vi "niRFUtil RFHS Channelizer CreateChannelizer CSG phaseII.vi"(0 "Channelizer Spec":T3={"freq in Hz"=TRUE, "Filter Type Hint"=enum."Auto", "Hint Value"=0.0, "Channels"=[]} {"Channels"."Flags" items=["None"=0, "Force Fractional"=1, "Use Multistage"=2, "Use Pretrigger Data "=256, "Frequency Shift Only"=4]; "Channels"."fs" format="%#_8p"; "Channels"."fc" format="%#_6p"; "Channels"."stopBW" format="%#_6p"; "Channels"."passBW" format="%#_6p"; "Hint Value" format="%#_8p"}, 1 "Type":T1, 2 "Benchmark Task":T8, 3 "Replace Filter Data":bool, 5 "fs [Hz]":dbl=1000000000.0 format="%#_6p", 7 "Mode":T2, 9 "Buffer Size (s)":dbl=0.003 format="%#_6p", 11 "error in (no error)":errorcluster, 13 "User Filter Spec":T7) -> (4 "Channelizer Ref":refnum<data-value>, 15 "error out":errorcluster)   [LabVIEW 2015, in "niRFUtil.lvlib"]
uses:
  niRFUtil.lvlib
  Utilities/Benchmark/niRFUtil RFHS Benchmark Task.ctl
  Utilities/niRFUtil RFHS Util User Filter Specification.ctl
  Includes/niRFUtil RFHS Channelizer ChannelSpecification.ctl
  Includes/niRFUtil RFHS Channelizer FilterTypeHint.ctl
  Includes/niRFUtil RFHS Channelizer ChannelSpecificationBase.ctl
  Includes/niRFUtil RFHS Channelizer ChannelFlags.ctl
  Includes/niRFUtil RFHS Channelizer ChannelizerBufferingMode.ctl
  Includes/niRFUtil RFHS Channelizer ChannelizerInfo CSG.ctl
  Includes/niRFUtil RFHS Channelizer FilterRef.ctl
  Utilities/Data FIFO/niRFUtil RFHS FIFO Reference.ctl
  Utilities/Data FIFO/niRFUtil RFHS FIFO.ctl
  Includes/niRFUtil RFHS Channelizer ChannelizerType.ctl
  Includes/niRFUtil RFHS Channelizer ChannelizerFlags.ctl
  Includes/niRFUtil RFHS Channelizer FilterSpecification.ctl
panel:
  in  "Inital Phase":dbl
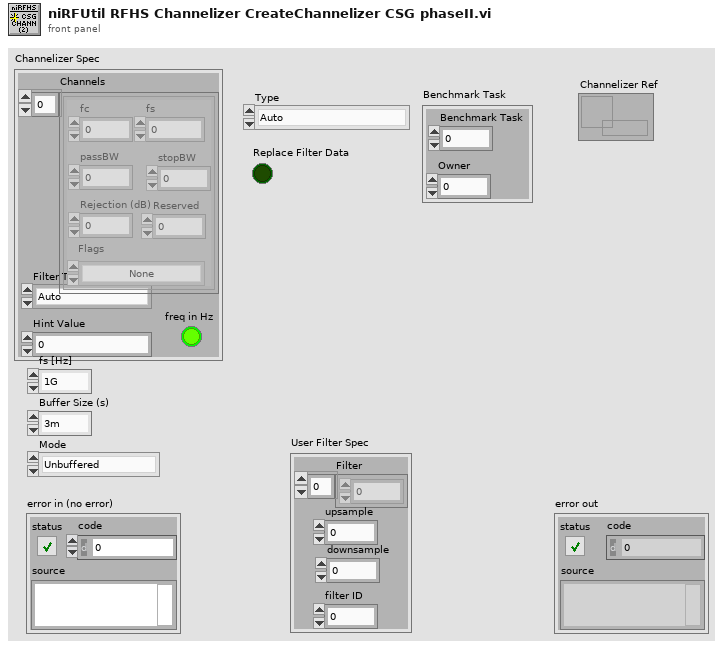
[diagram p1: front panel]
types:
  T1 = typedef "niRFUtil.lvlib/niRFUtil RFHS Channelizer ChannelizerType.ctl" = enum32{"Auto", "Frequency Shift Only", "Resampler Only"}
  T2 = typedef "niRFUtil.lvlib/niRFUtil RFHS Channelizer ChannelizerBufferingMode.ctl" = enum32{"Unbuffered", "Finite", "Continuous"}
  T3 = typedef "niRFUtil.lvlib/niRFUtil RFHS Channelizer ChannelSpecification.ctl" = cluster{"freq in Hz":bool, "Filter Type Hint":T4, "Hint Value":dbl, "Channels":T5[]}
  T4 = typedef "niRFUtil.lvlib/niRFUtil RFHS Channelizer FilterTypeHint.ctl" = enum16{"Auto", "FFT (LTE)", "FFT (WiFi)", "FFT (custom)"}
  T5 = typedef "niRFUtil.lvlib/niRFUtil RFHS Channelizer ChannelSpecificationBase.ctl" = cluster{"fc":dbl, "fs":dbl, "passBW":dbl, "stopBW":dbl, "Rejection (dB)":dbl, "Flags":T6, "Reserved":i32}
  T6 = typedef "niRFUtil.lvlib/niRFUtil RFHS Channelizer ChannelFlags.ctl" = u32
  T7 = typedef "niRFUtil.lvlib/niRFUtil RFHS Util User Filter Specification.ctl" = cluster{"Filter":dbl[], "upsample":i32, "downsample":i32, "filter ID":i32}
  T8 = typedef "niRFUtil.lvlib/niRFUtil RFHS Benchmark Task.ctl" = cluster{"Benchmark Task":u64, "Owner":u32}
  T9 = typedef "niRFUtil.lvlib/niRFUtil RFHS Channelizer ChannelizerInfo CSG.ctl" = cluster{"Filter LVRef":T10, "Mode":T2, "History":csg[], "Buffer":csg[], "FIFO":T11, "History Len":u32, "Float Cache":csg[], "Double Cache":cdb[], "Type":T1, "Resample Phase":dbl, "fft1Descriptors":u64[], "fft2Descriptors":u64[], "FFT tBuf":csg[], "guardBandLen":i32, "FFT History":csg[], "FFT History Len":u32, "FFTInitDone":u32, "FFT Filter LVRefs":T10[], "FFT fc Offs":u32[], "fft2Sizes":u32[], "BufferW":u32[], "BufferR":u32[], "Buff Off":u32[], "Phase0 (fshift)":dbl[], "Phase (fshift)":dbl[], "fs phase step":dbl[], "Resample Step":dbl, "Flags":T13, "Reset Cnt":i64, "Filter Pass":u32, "Stages":variant[]}
  T10 = typedef "niRFUtil.lvlib/niRFUtil RFHS Channelizer FilterRef.ctl" = cluster{"Ref":u64, "GUID":u64, "Upsample":i32, "Downsample":i32, "Size":i32, "Num Taps":i32}
  T11 = typedef "niRFUtil.lvlib/niRFUtil RFHS FIFO Reference.ctl" = cluster{"Read Lock":refnum<data-value>, "Info":T12, "Write Lock":refnum<data-value>}
  T12 = typedef "niRFUtil.lvlib/niRFUtil RFHS FIFO.ctl" = cluster{"ID":u64, "Length":u32}
  T13 = typedef "niRFUtil.lvlib/niRFUtil RFHS Channelizer ChannelizerFlags.ctl" = u32
  T14 = enum32{"Reserved", "Rational", "Fine Tune", "Fractional", "Rational (user)", "Reserved 2", "Fractional (user)", "FFT Resampler"}
  T15 = typedef "niRFUtil.lvlib/niRFUtil RFHS Channelizer FilterSpecification.ctl" = cluster{"Type":enum32{"Reserved", "Rational", "Fine Tune", "Fractional", "Rational (user)", "Reserved 2", "Fractional (user)", "FFT Resampler"}, "Reserved":i32, "Spec":T5}
  T16 = enum32{"Reserved", "Rational", "Fine Tune", "Fractional", "Rational (user)", "Reserved 2", "Fractional (user)"}
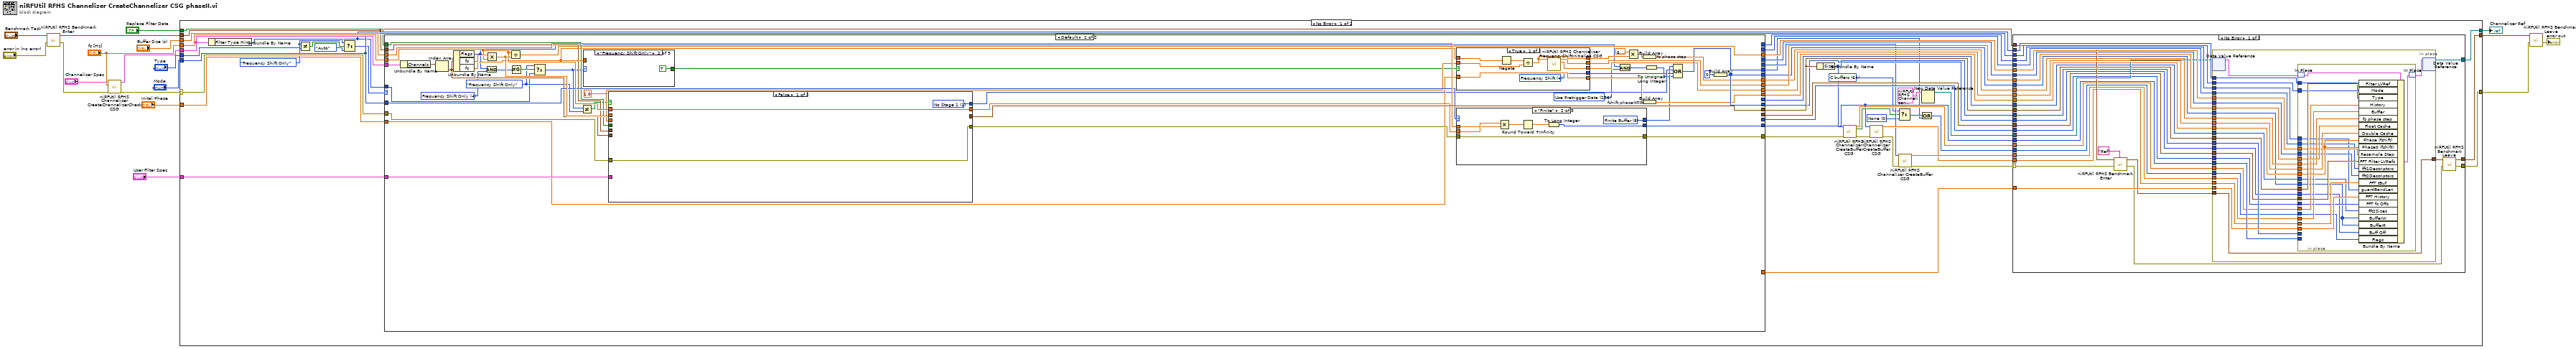
[diagram p0: block diagram]
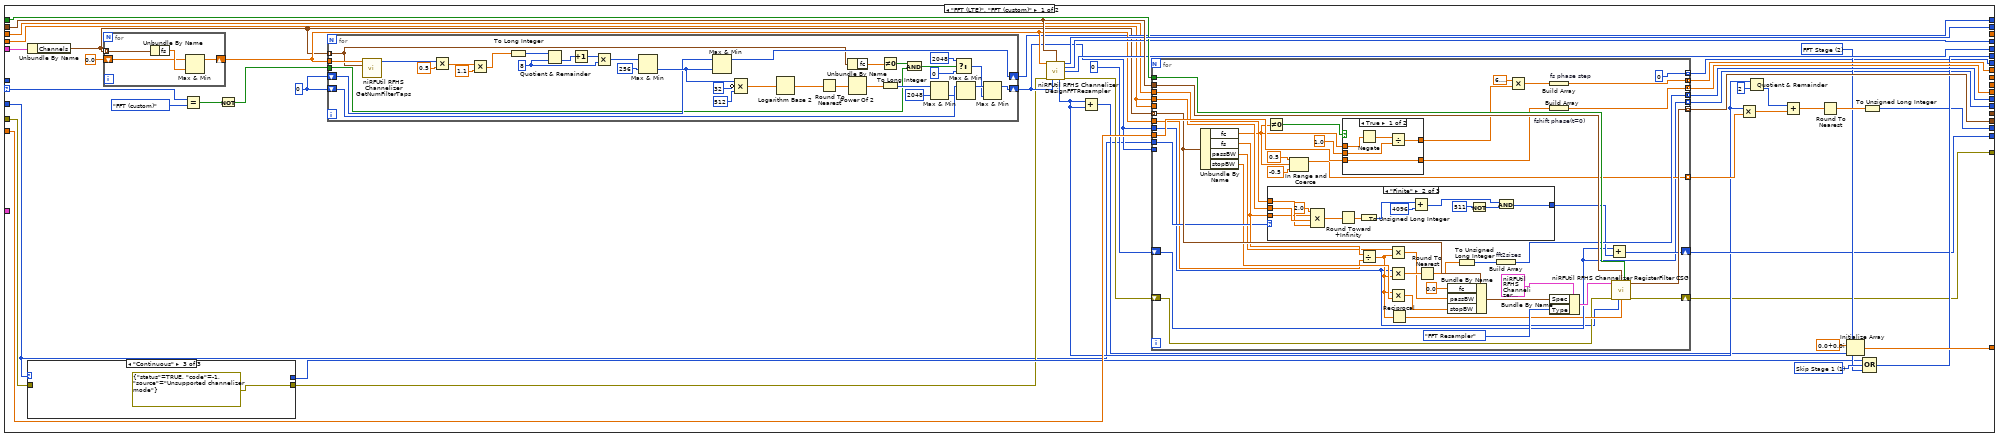
[diagram p3: hidden frame]
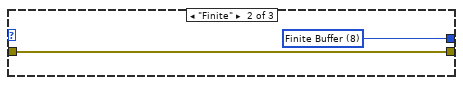
[diagram p8: hidden frame]
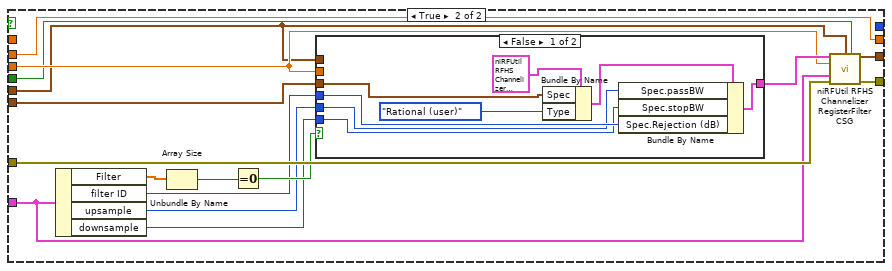
[diagram p10: hidden frame]
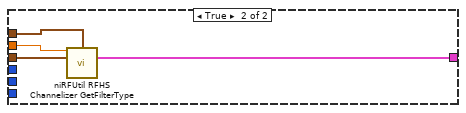
[diagram p11: hidden frame]
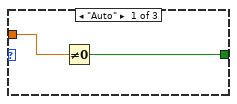
[diagram p12: hidden frame]
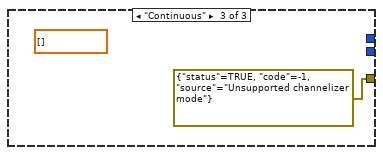
[diagram p15: hidden frame]
diagram:
  n1 = call "niRFUtil RFHS Benchmark Enter.vi"("error in (no error)"="error in (no error)", "Benchmark Task (Parent)"="Benchmark Task") -> ("error out"=w5:errorcluster, "Benchmark Task (Self)"=w7:T8)  [unwired: 8 in]
  n2 = call "niRFUtil RFHS Channelizer CreateChannelizerCheck CSG.vi"("Channel Spec"="Channelizer Spec", "fs [Hz]"="fs [Hz]", "error in (no error)"=w5) -> ("Channel Spec (out)"=w1:T3, "error out"=w4:errorcluster)  [unwired: 11 in]
  n3 = case shown="No Error" w4 {
    selector: w4 -> [w69 w404]
    tunnel: [w37 w404] -> w17
    tunnel: w1 -> [w19 _]
    tunnel: "fs [Hz]" -> [w62 _]
    tunnel: "User Filter Spec" -> [w68 _]
    tunnel: "Mode" -> [w61 _]
    tunnel: "Type" -> [w55 _]
    tunnel: w7 -> [w20 w403]
    tunnel: [w48 _] -> w11
    tunnel: "Buffer Size (s)" -> [w66 _]
    tunnel: "Inital Phase" -> [w43 _]
    tunnel: "Replace Filter Data" -> [w53 _]
    tunnel: [w47 w403] -> w6
    frame No Error {
      w22 = T13 64 items=["None"=0, "Skip Stage 1"=1, "FFT Stage"=2, "Frequency Shift"=4, "Finite Buffer"=8, "Reset"=16, "Input Len Estimate"=32, "C buffers"=64] ("t")
      w23 = T13 0 items=["None"=0, "Skip Stage 1"=1, "FFT Stage"=2, "Frequency Shift"=4, "Finite Buffer"=8, "Reset"=16, "Input Len Estimate"=32] ("Flags")
      n4 = Unbundle By Name(w19) -> ("Filter Type Hint"=w59:T4)
      n5 = Not Equal?(x=w55, y=niRFUtil_RFHS_Channelizer_ChannelizerType."Frequency Shift Only") -> (x != y?=w54:bool)
      n6 = Select(t=w59, s=w54, f=niRFUtil_RFHS_Channelizer_FilterTypeHint."Auto") -> (s? t:f=w40:T4)
      n7 = case shown="Default" w40 {
        selector: w40 -> [w159 _]
        tunnel: w69 -> [w154 w351]
        tunnel: w68 -> [_ w350]
        tunnel: [_ w349] -> w67
        tunnel: [w162 w347] -> w36
        tunnel: w66 -> [w173 w346]
        tunnel: [_ w318] -> w65
        tunnel: [_ w317] -> w64
        tunnel: [_ w325] -> w63
        tunnel: w62 -> [w172 w342]
        tunnel: w19 -> [w182 w326]
        tunnel: w61 -> [w161 w341]
        tunnel: w20 -> [w200 w340]
        tunnel: [w199 _] -> w58
        tunnel: [w198 _] -> w57
        tunnel: [w176 _] -> w56
        tunnel: w55 -> [_ w307]
        tunnel: w53 -> [w197 w339]
        tunnel: [w196 _] -> w52
        tunnel: [w169 w338] -> w32
        tunnel: [w195 _] -> w27
        tunnel: [w174 _] -> w46
        tunnel: [w194 _] -> w38
        tunnel: [w168 w332] -> w45
        tunnel: [w193 _] -> w39
        tunnel: [w170 w332] -> w44
        tunnel: w43 -> [w192 w335]
        tunnel: [w184 w330] -> w42
        tunnel: [w183 w328] -> w41
        tunnel: [w179 w319] -> w24
        frame "FFT (LTE)", "FFT (custom)" {
          w156 = 0
          w180 = T13 2 items=["None"=0, "Skip Stage 1"=1, "FFT Stage"=2, "Frequency Shift"=4] ("Flags")
          w181 = T13 1 items=["None"=0, "Skip Stage 1"=1, "FFT Stage"=2, "Frequency Shift"=4] ("Flags")
          n8 = Unbundle By Name(w182) -> ("Channels"=w155:T5[])
          n9 = case shown="\"Continuous\"" w161 {
            tunnel: w154 -> [w301 w303 _]
            tunnel: [w301 w303 errorcluster {"status"=TRUE, "code"=-1, "source"="Unsupported channelizer mode"} ("error out")] -> w164
            tunnel: [_ w302 _] -> w167
            frame "Unbuffered" {
            }
            frame "Finite" {
              w302 = T13 8 items=["None"=0, "Skip Stage 1"=1, "FFT Stage"=2, "Frequency Shift"=4, "Finite Buffer"=8] ("Flags")
            }
            frame "Continuous" {
            }
          }
          n10 = for {
            tunnel: w155 -> [w265] mode=indexing
            shift-right: [w263] -> w177
            shift-left: 0.0 -> [w262]
            n11 = Unbundle By Name(w265) -> ("fs"=w264:dbl)
            n12 = Max & Min(x=w262, y=w264) -> (max(x,y)=w263:dbl)  [unwired: 1 out]
          }
          n13 = Equal?(x=w159, y=niRFUtil_RFHS_Channelizer_FilterTypeHint."FFT (custom)") -> (x = y?=w158:bool)
          n14 = Not(x=w158) -> (.not. x?=w157:bool)
          n15 = for {
            tunnel: w155 -> [w275] mode=indexing
            shift-right: [w266] -> w175
            shift-left: w156 -> [w282]
            tunnel: w177 -> [w281]
            shift-right: [w277] -> w176
            shift-left: w156 -> [w278]
            tunnel: w157 -> [w272]
            w291 = 8 ("y")
            n16 = call "niRFUtil RFHS Channelizer GetNumFilterTaps.vi"("fs"=w281, "Channel Specification"=w275) -> ("#Filter Taps"=w280:i32)  [unwired: 13 in]
            n17 = Multiply(x=w280, y=0.5) -> (x*y=w284:dbl)
            n18 = Multiply(x=w284, y=1.1) -> (x*y=w286:dbl)
            n19 = To Long Integer(number=w286) -> (32bit integer=w288:i32)
            n20 = Quotient & Remainder(x=w288, y=w291) -> (floor(x/y)=w289:i32)  [unwired: 1 out]
            n21 = Increment(x=w289) -> (x+1=w290:i32)
            n22 = Multiply(x=w290, y=w291) -> (x*y=w292:i32)
            n23 = Max & Min(x=w292, y=256) -> (min(x,y)=w279:i32)  [unwired: 1 out]
            n24 = Max & Min(x=w278, y=w279) -> (max(x,y)=w277:i32)  [unwired: 1 out]
            n25 = Compound Arithmetic op=MULTIPLY(w279, invert 32 ("value"), 512 ("value")) -> (w295:dbl)
            n26 = Logarithm Base 2(1:w295) -> (0:w296:dbl)
            n27 = Round To Nearest(number=w296) -> (nearest integer value=w297:dbl)
            n28 = Unbundle By Name(w275) -> ("fc"=w274:dbl)
            n29 = Power Of 2(x=w297) -> (2^x=w298:dbl)
            n30 = Not Equal To 0?(x=w274) -> (x != 0?=w273:bool)
            n31 = To Long Integer(number=w298) -> (32bit integer=w299:i32)
            n32 = And(x=w273, y=w272) -> (x .and. y?=w270:bool)
            n33 = Max & Min(x=w299, y=2048) -> (min(x,y)=w276:i32)  [unwired: 1 out]
            n34 = Select(t=2048 ("Len Hint"), s=w270, f=0 ("Len Hint")) -> (s? t:f=w267:i32)
            n35 = Max & Min(x=w282, y=w276) -> (max(x,y)=w268:i32)  [unwired: 1 out]
            n36 = Max & Min(x=w268, y=w267) -> (max(x,y)=w266:i32)  [unwired: 1 out]
          }
          n37 = call "niRFUtil RFHS Channelizer DesignFFTResampler.vi"("Channel fs"=w177, "Benchmark Task"=w200, "error in (no error)"=w164, "fft2Size"=w175) -> ("fft1Descriptors"=w198:u64[], "fft2Descriptors"=w193:u64[], "Buffer Size"=w195:i32, "fft1Size"=w166:i32, "error out"=w163:errorcluster)  [unwired: 7 in]
          n38 = Add(x=w166, y=w166) -> (x+y=w165:i32)
          n39 = for {
            tunnel: w200 -> [w243]
            tunnel: [w224] -> w199 mode=indexing
            tunnel: w197 -> [w242]
            tunnel: [w241] -> w194 mode=concatenating
            tunnel: w192 -> [w239]
            tunnel: [w223] -> w185 mode=indexing
            tunnel: [w230] -> w184 mode=concatenating
            tunnel: [w229] -> w183 mode=concatenating
            tunnel: w155 -> [w228] mode=indexing
            tunnel: w172 -> [_]
            tunnel: w175 -> [w202]
            tunnel: w177 -> [w208]
            tunnel: w175 -> [_]
            tunnel: w173 -> [w220]
            tunnel: w172 -> [w219]
            tunnel: w161 -> [w217]
            tunnel: [w214] -> w170 mode=indexing
            shift-right: [w216] -> w169
            shift-left: u32 0 -> [w214]
            tunnel: [u32 0] -> w168 mode=indexing
            shift-right: [w204] -> w162
            shift-left: w163 -> [w205]
            n40 = Unbundle By Name(w228) -> ("fc"=w201:dbl, "fs"=w218:dbl, "passBW"=w212:dbl, "stopBW"=w210:dbl)
            n41 = Not Equal To 0?(x=w201) -> (x != 0?=w203:bool)
            n42 = case shown="\"Finite\"" w217 {
              tunnel: w220 -> [_ w255 _]
              tunnel: w219 -> [_ w256 _]
              tunnel: [_ w247 _] -> w215
              tunnel: w218 -> [_ w252 _]
              frame "Unbuffered" {
              }
              frame "Finite" {
                n43 = Compound Arithmetic op=MULTIPLY(2.0 ("value"), w252, w256, w255) -> (w254:dbl)
                n44 = Round Toward +Infinity(x=w254) -> (ceil(x): smallest int >= x=w253:dbl)
                n45 = To Unsigned Long Integer(number=w253) -> (unsigned 32bit integer=w251:u32)
                n46 = Add(x=w251, y=u32 4096) -> (x+y=w249:u32)
                n47 = Not(x=u32 511 ("y")) -> (.not. x?=w246:u32)
                n48 = And(x=w249, y=w246) -> (x .and. y?=w247:u32)
              }
              frame "Continuous" {
              }
            }
            n49 = In Range and Coerce(upper limit=0.5, x=w201, lower limit=-0.5) -> (coerced(x)=w223:dbl)  [unwired: 1 out]
            n50 = case shown="True" w203 {
              tunnel: [w260 _] -> w227
              tunnel: 1.0 ("t") -> [w261 _]
              tunnel: w239 -> [w259 _]
              tunnel: [w259 _] -> w231
              tunnel: w201 -> [w258 _]
              frame True {
                n51 = Negate(x=w258) -> (-x=w257:dbl)
                n52 = Divide(x=w257, y=w261) -> (x/y=w260:dbl)
              }
              frame False {
              }
            }
            n53 = Divide(x=w218, y=w208) -> (x/y=w207:dbl)
            n54 = Multiply(x=w212, y=w207) -> (x*y=w211:dbl)
            n55 = Multiply(x=w202, y=w207) -> (x*y=w222:dbl)
            n56 = Multiply(x=w207, y=w210) -> (x*y=w209:dbl)
            n57 = Reciprocal(x=w207) -> (1/x=w206:dbl)
            n58 = Round To Nearest(number=w222) -> (nearest integer value=w221:dbl)
            n59 = Bundle By Name(cluster=w228, "fc"=0.0, "passBW"=w211, "stopBW"=w209) -> (w244:T5)
            n60 = To Unsigned Long Integer(number=w221) -> (unsigned 32bit integer=w235:u32)
            n61 = Build Array "fft2sizes"(w235) -> (w241:u32[])
            n62 = Multiply(x=6.283185307179586, y=w227) -> (x*y=w225:dbl)
            n63 = Build Array "fs phase step"(w225) -> (w229:dbl[])
            n64 = Build Array "fshift phase(t=0)"(w231) -> (w230:dbl[])
            n65 = Bundle By Name(cluster=T15 {"Type"=enum."Rational", "Reserved"=0, "Spec"={"fc"=0.0, "fs"=0.0, "passBW"=0.0, "stopBW"=0.0, "Rejection (dB)"=0.0, "Flags"=0, "Reserved"=0}} ("Filter Spec"), "Spec"=w244, "Type"=T14."FFT Resampler") -> (w236:T15)
            n66 = Add(x=w214, y=w215) -> (x+y=w216:u32)
            n67 = call "niRFUtil RFHS Channelizer RegisterFilter CSG.vi"("Filter Spec"=w236, "Benchmark Task"=w243, "Replace Filter Data"=w242, "error in (no error)"=w205, "Len Hint"=w202, "Filter Scaling"=w206) -> ("Filter LVRef"=w224:T10, "error out"=w204:errorcluster)  [unwired: 8 in]
          }
          n68 = Multiply(x=w166, y=w185) -> (x*y=w188:dbl[])
          n69 = Quotient & Remainder(x=w166, y=2) -> (floor(x/y)=w189:i32)  [unwired: 1 out]
          n70 = Add(x=w189, y=w188) -> (x+y=w187:dbl[])
          n71 = Round To Nearest(number=w187) -> (nearest integer value=w186:dbl[])
          n72 = Initialize Array(csg 0.0+0.0i ("element"), w165) -> (w196:csg[])
          n73 = Compound Arithmetic op=OR(w167, w181, w180) -> (w179:T13)
          n74 = To Unsigned Long Integer(number=w186) -> (unsigned 32bit integer=w174:u32[])
        }
        frame Default {
          w311 = T6 4 items=["None"=0, "Force Fractional"=1, "Use Multistage"=2, "Use Pretrigger Data "=256, "Frequency Shift Only"=4] ("y")
          w315 = T6 256 items=["None"=0, "Force Fractional"=1, "Use Multistage"=2, "Use Pretrigger Data "=256] ("y")
          w308 = niRFUtil_RFHS_Channelizer_ChannelizerType."Frequency Shift Only" ("y")
          w337 = 1.0 ("t")
          n75 = Unbundle By Name(w326) -> ("Channels"=w327:T5[])
          n76 = Index Array(array=w327) -> (element=w312:T5)  [unwired: 1 in]
          n77 = Unbundle By Name(w312) -> ("Flags"=w305:T6, "fs"=w345:dbl, "fc"=w336:dbl)
          n78 = And(x=w305, y=w311) -> (x .and. y?=w310:T6)
          n79 = Multiply(x=w345, y=w342) -> (x*y=w343:dbl)
          n80 = Divide(x=w342, y=w343) -> (x/y=w325:dbl)
          n81 = Not Equal To 0?(x=w310) -> (x != 0?=w309:bool)
          n82 = Select(t=w308, s=w309, f=w307) -> (s? t:f=w306:T1)
          n83 = Not Equal?(x=w306, y=w308) -> (x != y?=w331:bool)
          n84 = case shown="\"Frequency Shift Only\"" w306 {
            tunnel: [w392 TRUE _] -> w329
            tunnel: w336 -> [w391 _ _]
            frame "Auto" {
              n85 = Not Equal To 0?(x=w391) -> (x != 0?=w392:bool)
            }
            frame "Frequency Shift Only" {
            }
            frame "Resampler Only" {
            }
          }
          n86 = case shown="False" w331 {
            tunnel: w351 -> [w362 w378]
            tunnel: w350 -> [_ w372]
            tunnel: [_ w377] -> w349
            tunnel: [w362 w376] -> w348
            tunnel: w340 -> [_ w363]
            tunnel: w312 -> [_ w374]
            tunnel: w337 -> [_ w367]
            tunnel: w343 -> [_ w375]
            tunnel: [w361 w375] -> w344
            tunnel: w342 -> [w361 _]
            tunnel: w339 -> [_ w364]
            tunnel: [w360 _] -> w321
            frame False {
              w360 = T13 1 items=["None"=0, "No Stage 1"=1, "FFT Stage"=2, "Frequency Shift"=4] ("Flags")
            }
            frame True {
              n87 = Unbundle By Name(w372) -> ("Filter"=w371:dbl[], "filter ID"=w368:i32, "upsample"=w366:i32, "downsample"=w365:i32)
              n88 = Array Size(array=w371) -> (size(s)=w370:i32)
              n89 = Equal To 0?(x=w370) -> (x = 0?=w369:bool)
              n90 = case shown="False" w369 {
                tunnel: w374 -> [w385 w390]
                tunnel: [w382 w389] -> w373
                tunnel: w367 -> [_ w388]
                tunnel: w368 -> [w381 _]
                tunnel: w366 -> [w380 _]
                tunnel: w365 -> [w379 _]
                tunnel: w363 -> [_ w387]
                frame False {
                  n91 = Bundle By Name(cluster=T15 {"Type"=enum."Reserved", "Reserved"=0, "Spec"={"fc"=0.0, "fs"=0.0, "passBW"=0.0, "stopBW"=0.0, "Rejection (dB)"=0.0, "Flags"=0, "Reserved"=0}} ("Filter Spec"), "Spec"=w385, "Type"=T16."Rational (user)") -> (w383:T15)
                  n92 = Bundle By Name(cluster=w383, "Spec.passBW"=w380, "Spec.stopBW"=w379, "Spec.Rejection (dB)"=w381) -> (w382:T15)
                }
                frame True {
                  n93 = call "niRFUtil RFHS Channelizer GetFilterType.vi"("fs"=w388, "Benchmark Task"=w387, "Channel Specification"=w390) -> ("Filter Spec"=w389:T15)  [unwired: 9 in, 3 out]
                }
              }
              n94 = call "niRFUtil RFHS Channelizer RegisterFilter CSG.vi"("Filter Spec"=w373, "Benchmark Task"=w363, "Replace Filter Data"=w364, "fs"=w367, "User Filter Spec"=w372, "error in (no error)"=w378) -> ("Filter LVRef"=w377:T10, "error out"=w376:errorcluster)  [unwired: 8 in]
            }
          }
          n95 = case shown="True" w329 {
            tunnel: [w354 _] -> w323
            tunnel: w337 -> [w359 _]
            tunnel: w335 -> [w358 _]
            tunnel: [w358 _] -> w334
            tunnel: w336 -> [w357 _]
            tunnel: [w355 _] -> w320
            tunnel: [w353 _] -> w318
            tunnel: [w352 _] -> w317
            frame True {
              w355 = T13 4 items=["None"=0, "No Stage 1"=1, "FFT Stage"=2, "Frequency Shift"=4] ("Flags")
              n96 = Negate(x=w357) -> (-x=w356:dbl)
              n97 = Divide(x=w356, y=w359) -> (x/y=w354:dbl)
              n98 = call "niRFUtil RFHS Channelizer FrequencyShiftInitialize CSG.vi"("fc"=w354) -> ("Float Cache"=w353:csg[], "Double Cache"=w352:cdb[])  [unwired: 13 in]
            }
            frame False {
            }
          }
          n99 = case shown="\"Finite\"" w341 {
            tunnel: w348 -> [w394 w401 _]
            tunnel: [w394 w401 errorcluster {"status"=TRUE, "code"=-1, "source"="Unsupported channelizer mode"} ("error out")] -> w347
            tunnel: w346 -> [_ w399 _]
            tunnel: w344 -> [_ w400 _]
            tunnel: [_ w396 _] -> w338
            tunnel: [_ w395 _] -> w316
            frame "Unbuffered" {
            }
            frame "Finite" {
              w395 = T13 8 items=["None"=0, "Skip Stage 1"=1, "FFT Stage"=2, "Frequency Shift"=4, "Finite Buffer"=8] ("Flags")
              n100 = Multiply(x=w400, y=w399) -> (x*y=w398:dbl)
              n101 = Round Toward +Infinity(x=w398) -> (ceil(x): smallest int >= x=w397:dbl)
              n102 = To Long Integer(number=w397) -> (32bit integer=w396:i32)
            }
            frame "Continuous" {
              (unwired) csg[] []
            }
          }
          n103 = And(x=w305, y=w315) -> (x .and. y?=w314:T6)
          n104 = Multiply(x=6.283185307179586, y=w323) -> (x*y=w322:dbl)
          n105 = Build Array "fs phase step"(w322) -> (w328:dbl[])
          n106 = Build Array "fshift phase(t=0)"(w334) -> (w330:dbl[])
          n107 = To Unsigned Long Integer(number=w314) -> (unsigned 32bit integer=w313:T6)
          n108 = Compound Arithmetic op=OR(w316, w321, w320, w313) -> (w319:T13)
          n109 = Build Array(u32 0) -> (w332:u32[])
        }
      }
      n110 = Unbundle By Name(w67) -> ("Size"=w35:i32)
      n111 = call "niRFUtil RFHS Channelizer CreateBuffer CSG.vi"("Size"=w35, "error in (no error)"=w36) -> ("Buffer"=w34:csg[], "Embedded?"=w26:bool, "error out"=w33:errorcluster)  [unwired: 11 in]
      n112 = call "niRFUtil RFHS Channelizer CreateBuffer CSG.vi"("Size"=w32, "error in (no error)"=w33) -> ("Buffer"=w31:csg[], "error out"=w30:errorcluster)  [unwired: 11 in, 1 out]
      n113 = Select(t=w22, s=w26, f=w23) -> (s? t:f=w25:T13)
      n114 = call "niRFUtil RFHS Channelizer CreateBuffer CSG.vi"("Size"=w27, "error in (no error)"=w30) -> ("Buffer"=w28:csg[], "error out"=w29:errorcluster)  [unwired: 11 in, 1 out]
      n115 = Or(x=w25, y=w24) -> (x .or. y?=w21:T13)
      n116 = New Data Value Reference(data value=T9 {"Filter LVRef"={"Ref"=0, "GUID"=0, "Upsample"=0, "Downsample"=0, "Size"=0, "Num Taps"=0}, "Mode"=enum."Unbuffered", "History"=[], "Buffer"=[], "FIFO"={"Read Lock"=refnum, "Info"={"ID"=0, "Length"=0}, "Write Lock"=refnum}, "History Len"=0, "Float Cache"=[], "Double Cache"=[], "Type"=enum."Auto", "Resample Phase"=0.0, "fft1Descriptors"=[], "fft2Descriptors"=[], "FFT tBuf"=[], "guardBandLen"=0, "FFT History"=[], "FFT History Len"=0, "FFTInitDone"=0, "FFT Filter LVRefs"=[], "FFT fc Offs"=[], "fft2Sizes"=[], "BufferW"=[], "BufferR"=[], "Buff Off"=[], "Phase0 (fshift)"=[], "Phase (fshift)"=[], "fs phase step"=[], "Resample Step"=0.0, "Flags"=0, "Reset Cnt"=0, "Filter Pass"=0, "Stages"=[]} ("Info")) -> (data value reference=w49:refnum<data-value>)  [unwired: 1 in, 1 out]
      n117 = case shown="No Error" w29 {
        selector: w29 -> [w72 w152]
        tunnel: w67 -> [w102 _]
        tunnel: w65 -> [w101 _]
        tunnel: w64 -> [w100 _]
        tunnel: w63 -> [w99 _]
        tunnel: w61 -> [w98 _]
        tunnel: w58 -> [w97 _]
        tunnel: w57 -> [w96 _]
        tunnel: w56 -> [w95 _]
        tunnel: w55 -> [w94 _]
        tunnel: w52 -> [w93 _]
        tunnel: w49 -> [w92 _]
        tunnel: [w91 _] -> w48
        tunnel: w20 -> [w90 w153]
        tunnel: [w89 w153] -> w47
        tunnel: w35 -> [w88 _]
        tunnel: w34 -> [w87 _]
        tunnel: w32 -> [w86 _]
        tunnel: w31 -> [w85 _]
        tunnel: w28 -> [w84 _]
        tunnel: w46 -> [w83 _]
        tunnel: w45 -> [w82 _]
        tunnel: w44 -> [w81 _]
        tunnel: w42 -> [w80 _]
        tunnel: w41 -> [w79 _]
        tunnel: w39 -> [w78 _]
        tunnel: w38 -> [w77 _]
        tunnel: w21 -> [w76 _]
        tunnel: [w70 w152] -> w37
        frame No Error {
          n118 = call "niRFUtil RFHS Benchmark Enter.vi"("ID"="Ref", "error in (no error)"=w72, "Benchmark Task (Parent)"=w90) -> ("error out"=w71:errorcluster, "Benchmark Task (Self)"=w74:T8)  [unwired: 7 in]
          n119 = in-place {
            in-place-border: w102 -> [w128]
            in-place-border: w101 -> [w127]
            in-place-border: w100 -> [w126]
            in-place-border: w79 -> [w125]
            in-place-border: w80 -> [w124]
            in-place-border: w99 -> [w123]
            in-place-border: w98 -> [w122]
            in-place-border: w97 -> [w121]
            in-place-border: w96 -> [w120]
            in-place-border: w78 -> [w119]
            in-place-border: w95 -> [w118]
            in-place-border: w94 -> [w117]
            in-place-border: w93 -> [w116]
            in-place-border: [w115] -> w73
            in-place-border: w74 -> [w115]
            in-place-border: w88 -> [w112]
            in-place-border: w86 -> [w111]
            in-place-border: w85 -> [w110]
            in-place-border: w87 -> [w109]
            in-place-border: w84 -> [w108]
            in-place-border: w83 -> [w107]
            in-place-border: w77 -> [w106]
            in-place-border: w82 -> [w105]
            in-place-border: w81 -> [w104]
            in-place-border: w76 -> [w103]
            n120 = in-place-dvr #1(w92) -> (w114:T9)  [unwired: 1 out]
            n121 = in-place {
              in-place-border: w128 -> [w151]
              in-place-border: w127 -> [w150]
              in-place-border: w126 -> [w149]
              in-place-border: w125 -> [w148]
              in-place-border: w124 -> [w147]
              in-place-border: w123 -> [w146]
              in-place-border: w122 -> [w145]
              in-place-border: w121 -> [w144]
              in-place-border: w120 -> [w143]
              in-place-border: w119 -> [w142]
              in-place-border: w118 -> [w141]
              in-place-border: w117 -> [w140]
              in-place-border: w116 -> [w139]
              in-place-border: w112 -> [_]
              in-place-border: w111 -> [_]
              in-place-border: w110 -> [w136]
              in-place-border: w109 -> [w135]
              in-place-border: w108 -> [w134]
              in-place-border: w107 -> [w133]
              in-place-border: w106 -> [w132]
              in-place-border: w105 -> [w131]
              in-place-border: w104 -> [w130]
              in-place-border: w103 -> [w129]
              n122 = in-place-match #2(w114) -> (w137:T9)
              n123 = Bundle By Name(cluster=w137, "Filter LVRef"=w151, "Mode"=w145, "Type"=w140, "History"=w135, "Buffer"=w136, "fs phase step"=w148, "Float Cache"=w150, "Double Cache"=w149, "Phase (fshift)"=w147, "Phase0 (fshift)"=w147, "Resample Step"=w146, "FFT Filter LVRefs"=w144, "fft1Descriptors"=w143, "fft2Descriptors"=w142, "FFT tBuf"=w134, "guardBandLen"=w141, "FFT History"=w139, "FFT fc Offs"=w133, "fft2Sizes"=w132, "BufferW"=w131, "BufferR"=w131, "Buff Off"=w130, "Flags"=w129) -> (w138:T9)
              n124 = in-place-match #2(w138) -> (w113:T9)
            }
            n125 = in-place-dvr #1(w113) -> (w91:refnum<data-value>)  [unwired: 1 out]
          }
          n126 = call "niRFUtil RFHS Benchmark Leave.vi"("error in (no error)"=w71, "Benchmark Task Self"=w73) -> ("error out"=w70:errorcluster, "Benchmark Task Owner"=w89:T8)  [unwired: 8 in]
        }
        frame Error {
        }
      }
    }
    frame Error {
    }
  }
  "Channelizer Ref" <- w11
  n127 = call "niRFUtil RFHS Benchmark Leave.vi"("error in (no error)"=w17, "Benchmark Task Self"=w6) -> ("error out"=→"error out":errorcluster)  [unwired: 8 in, 1 out]
